vi "number_to_binary.vi"() -> ()   [LabVIEW 2020]
uses:
  <vilib>/MakerHub/LINX/Public/Peripherals/Digital/Digital Read 1 Chan.vi
  <vilib>/MakerHub/LINX/Public/Peripherals/Digital/Digital Write N Chans.vi
  <vilib>/MakerHub/LINX/Public/Peripherals/Digital/Digital Read N Chans.vi
  <vilib>/MakerHub/LINX/Private/Local IO/LinxDigitalWrite.vi
  <vilib>/MakerHub/LINX/Public/Utilities/Check Channel.vi
  <vilib>/MakerHub/LINX/Private/Local IO/LinxDigitalRead.vi
  <vilib>/MakerHub/LINX/Private/Local IO/Handle Errors.vi
  <vilib>/MakerHub/LINX/Public/Utilities/Open Local.vi
  <vilib>/MakerHub/LINX/Private/Utilties/Generate Error.vi
  <vilib>/MakerHub/LINX/LMH-LINX.lvlib
panel:
  in  "DO Channels":u8[](array[numeric])
  out "Boolean array":bool[](array[boolean])
  out "x+y":i16
  in  "DI Channel":u8=2
  in  "Stop Button":bool
  out "DI Value":bool
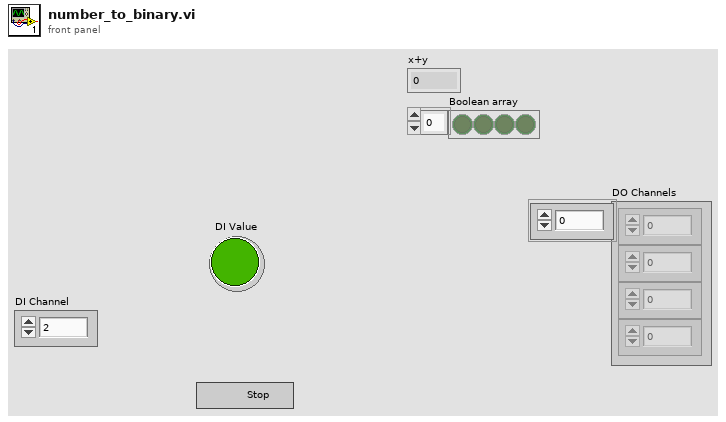
[diagram p1: front panel]
types:
  T1 = typedef "LMH-LINX.lvlib/LINX Ref.ctl" = cluster{"IO":T2, "Interface":T3, "LINX Device Config":T4}
  T2 = typedef "LMH-LINX.lvlib/Platform.ctl" = enum16{"Remote", "Local"}
  T3 = typedef "LMH-LINX.lvlib/Interface.ctl" = enum16{"Serial", "TCP"}
  T4 = typedef "LMH-LINX.lvlib/Device.lvlib/LINX Device Config.ctl" = cluster{"Interface":T3, "COM Port":refnum<visa-resource-name>, "TCP Configuration":T5, "Device Family":u8, "Device ID":u8, "Device Name":string, "TCP Ref":refnum<k5>, "Channels":T6}
  T5 = typedef "LMH-LINX.lvlib/Device.lvlib/TCP Config.ctl" = cluster{"IP Address":string, "Port":u16}
  T6 = typedef "LMH-LINX.lvlib/Channels.ctl" = cluster{"DI":u8[], "DO":u8[], "AI":u8[], "AO":u8[], "PWM":u8[], "QE":u8[], "UART":u8[], "I2C 2":u8[], "SPI":u8[], "CAN":u8[], "Servo":u8[], "AI Ref (V)":dbl, "AI Resolution (Bits)":u8, "AO Ref (V)":dbl, "AO Resolution (Bits)":u8}
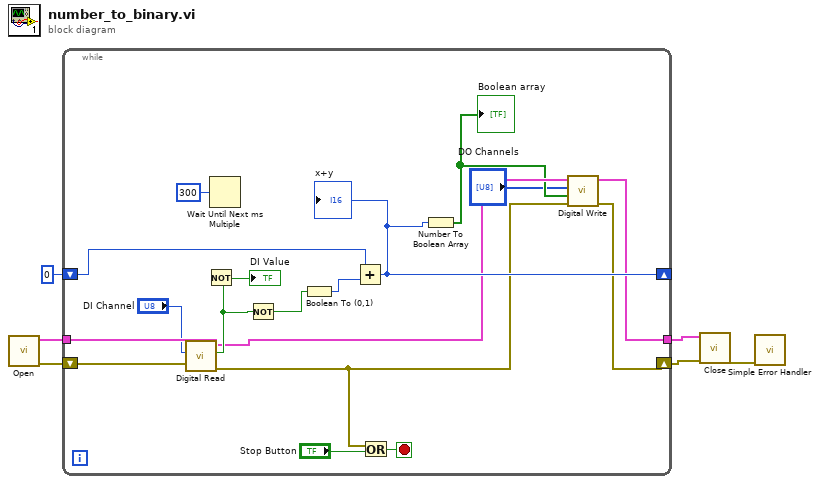
[diagram p0: block diagram]
diagram:
  n1 = call-poly <vilib>:"Open.vi"() -> ("Error Out"=w5:errorcluster, "LINX Resource"=w6:T1)  [unwired: 9 in, 1 out]
  n2 = while {
    tunnel: w6 -> [w22]
    tunnel: [w11] -> w4
    shift-right: [w9] -> w3
    shift-left: w5 -> [w21]
    shift-right: [w13] -> _
    shift-left: i16 0 -> [w19]
    stop <- w24 stop-if-true
    n3 = call-poly <vilib>:"Digital Read.vi"("Error In"=w21, "DI Channel"="DI Channel", "LINX Resource"=w22) -> ("Error Out"=w10:errorcluster, "DI Value"=w16:bool, "LINX Resource"=w12:T1)  [unwired: 6 in]
    n4 = Not(x=w16) -> (.not. x?=→"DI Value":bool)
    n5 = Wait Until Next ms Multiple(millisecond multiple=u32 300) -> ()  [unwired: 1 out]
    n6 = Not(x=w16) -> (.not. x?=w15:bool)
    n7 = Boolean To (0,1)(Boolean=w15) -> (0, 1=w20:i16)
    n8 = Add(x=w19, y=w20) -> (x+y=w13:i16)
    "x+y" <- w13
    n9 = Or(x=w10, y="Stop Button") -> (x .or. y?=w24:bool)
    n10 = Number To Boolean Array(number=w13) -> (Boolean array=w8:bool[])
    "Boolean array" <- w8
    n11 = call-poly <vilib>:"Digital Write.vi"("Error In"=w10, "Values"=w8, "DO Channels"="DO Channels", "LINX Resource"=w12) -> ("Error Out"=w9:errorcluster, "LINX Resource"=w11:T1)  [unwired: 6 in]
  }
  n12 = call <vilib>:"Close.vi"("Error In"=w3, "LINX Resource"=w4) -> ("Error Out"=w2:errorcluster)  [unwired: 9 in]
  n13 = call <vilib>:"Simple Error Handler.vi"("error in (no error)"=w2) -> ()  [unwired: 4 in, 5 out]
